vi "magnification.vi"(8 "error in (no error)":errorcluster, 11 "DAQOrcaFlash in":refnum<class "DAQOrcaFlash.lvclass">) -> (0 "error out":errorcluster, 3 "DAQOrcaFlash out":refnum<class "DAQOrcaFlash.lvclass">)   [LabVIEW 2012, in "DAQOrcaFlash.lvclass"]
uses:
  DAQOrcaFlash.lvclass
panel:
  out "slit width in object space":dbl[unit]
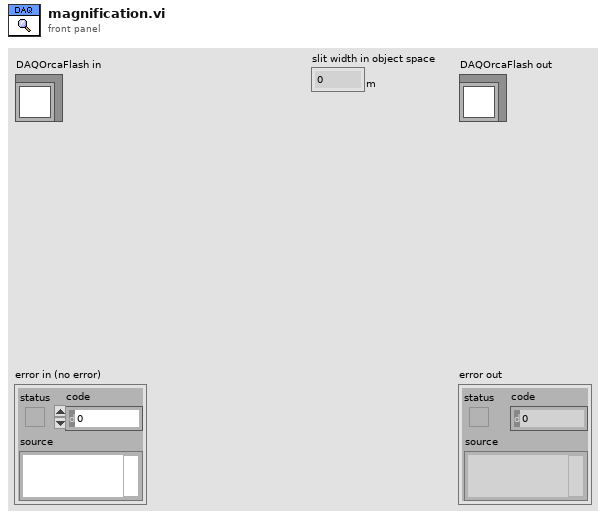
[diagram p1: front panel]
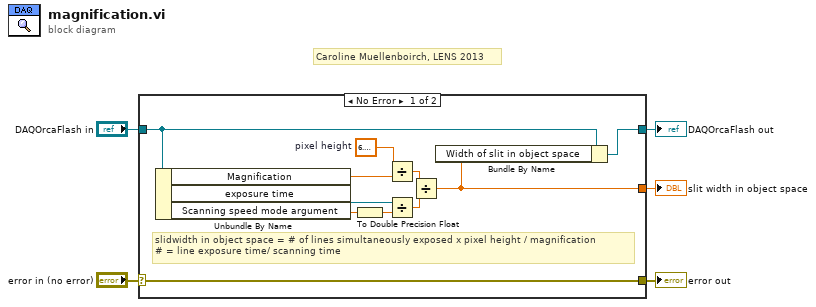
[diagram p0: block diagram]
diagram:
  # "Caroline Muellenboirch, LENS 2013"
  n1 = case shown="No Error" "error in (no error)" {
    selector: "error in (no error)" -> [w16 w18]
    tunnel: [w16 w18] -> w4
    tunnel: [w6 w17] -> w2
    tunnel: "DAQOrcaFlash in" -> [w9 w17]
    tunnel: [w7 _] -> w1
    frame No Error {
      w15 = dbl[unit] 6.5e-06  # pixel height
      # "slidwidth in object space = # of lines simultaneously exposed x pixel height / magnification\n# = line exposure time/ scanning time"
      n2 = Unbundle By Name(w9) -> ("Magnification"=w12:dbl, "exposure time"=w8:refnum<vi>, "Scanning speed mode argument"=w13:sgl[unit])
      n3 = To Double Precision Float(number=w13) -> (double precision float=w14:dbl[unit])
      n4 = Divide(x=w15, y=w12) -> (x/y=w11:dbl[unit])
      n5 = Divide(x=w8, y=w14) -> (x/y=w10:dbl)
      n6 = Divide(x=w11, y=w10) -> (x/y=w7:dbl[unit])
      n7 = Bundle By Name(cluster=w9, "Width of slit in object space"=w7) -> (w6:refnum<class "DAQOrcaFlash.lvclass">)
    }
    frame Error {
    }
  }
  "error out" <- w4
  "DAQOrcaFlash out" <- w2
  "slit width in object space" <- w1
